vi "LEBITVacuum.GetLogLocation.vi"(0 "i ref in":refnum<vi>, 5 "error in (no error)":errorcluster) -> (14 "i ref out":refnum<vi>, 16 "log location":string, 19 "error out 2":errorcluster)   [LabVIEW 2014, in "LEBITVacuum.lvlib"]
uses:
  LEBITVacuum.lvlib
  CSCore/BaseProcess/BaseProcess.lvlib
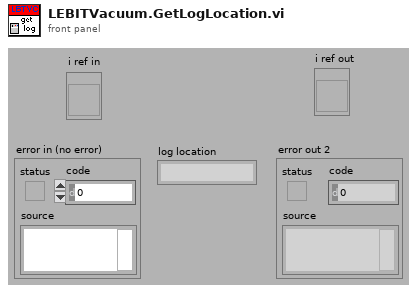
[diagram p1: front panel]
types:
  T1 = typedef "BaseProcess.lvlib/BaseProcess.i attribute.ctl" = cluster{"EventStatus":string, "EventError":i32, "PresetEvtWatchD":i32, "PresetPdcWatchD":i32, "EventTimeout":i32, "PeriodicInterval":i32, "Interface":string[], "Address":string[], "Special":string[], "PeriodicError":i32, "PeriodicStatus":string, "SuperProc":string, "Descriptors":T2[], "CaseRef":refnum<vi>, "PdcRef":refnum<vi>, "Thread Ref":refnum<vi>, "eventErrorID":i32, "eventStatusID":i32, "periodicErrorID":i32, "periodicStatusID":i32, "pdcCtrID":i32}
  T2 = typedef "BaseProcess.lvlib/BaseProcess.descriptor definition.ctl" = cluster{"selector":string, "descriptor":T3}
  T3 = typedef "BaseProcess.lvlib/BaseProcess.descriptor string definition.ctl" = string
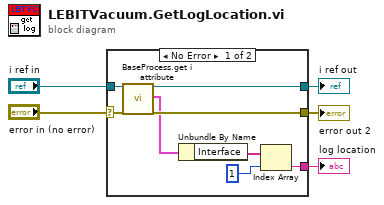
[diagram p0: block diagram]
diagram:
  n1 = case shown="No Error" "error in (no error)" {
    selector: "error in (no error)" -> [w6 w14]
    tunnel: "i ref in" -> [w13 w15]
    tunnel: [w12 w14] -> w2
    tunnel: [w11 w15] -> w3
    tunnel: [w7 _] -> w4
    frame No Error {
      n2 = call "BaseProcess.get i attribute.vi"("i ref in"=w13, "error in (no error)"=w6) -> ("i ref out"=w11:refnum<vi>, "i attribute"=w10:T1, "error out"=w12:errorcluster)  [unwired: 15 in]
      n3 = Unbundle By Name(w10) -> ("Interface"=w9:string[])
      n4 = Index Array(array=w9, index=1) -> (element=w7:string)
    }
    frame Error {
    }
  }
  "error out 2" <- w2
  "i ref out" <- w3
  "log location" <- w4
